vi "Create Reference.vi"(8 "Error In":errorcluster, 11 "Writer In":refnum<class "Writer.lvclass">) -> (0 "Error Out":errorcluster, 3 "Writer Out":refnum<data-value>)   [LabVIEW 2019, in "LabPack.lvlib" / "Writer.lvclass"]
doc: "Creates a Data Value Reference (DVR) of a Writer object. This facilitates a \"pass by reference\"-like approach to using the Writer class. Use this to ensure a single copy of a Writer object exists within an application."
uses:
  Writer.lvclass
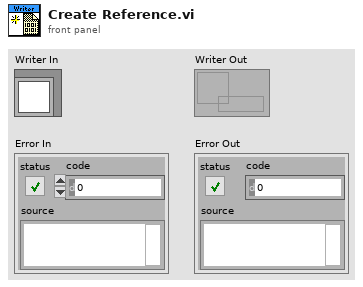
[diagram p1: front panel]
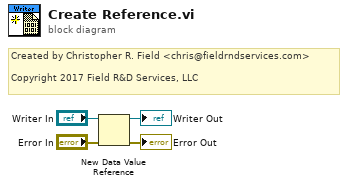
[diagram p0: block diagram]
diagram:
  # "Created by Christopher R. Field <chris@fieldrndservices.com>\n\nCopyright 2017 Field R&D Services, LLC"
  n1 = New Data Value Reference(data value="Writer In", error in="Error In") -> (data value reference=→"Writer Out":refnum<data-value>, error out=→"Error Out":errorcluster)
